vi "RT Loop - Acquisition and Logging.vi"(8 "error in (no error)":errorcluster, 9 "Acquisition and Logging Configuration":T1={"Data Rate (Hz)"=1.0, "Samples per Read"=0, "Number of Reads to Save"=0, "Data File Name"="", "TDMS Properties"=[], "Number of Channels"=4, "Channel Scale Array"=[0.0, 0.0, 0.0, 0.0], "Channel Names"=[], "Trigger - RMS Value"=0.0, "Trigger - Channel"=0, "Trigger - Time (Minute)"=0, "Enable RMS Trigger"=FALSE, "Enable Time Trigger"=FALSE, "Always Log"=FALSE}, 10 "Acquisition and Logging Queue":refnum<queue>, 11 "Message Queue":refnum<queue>) -> ()   [LabVIEW 2022 SP3]
uses:
  support/Message Queue/Message Cluster.ctl
  controls/Acquisition and Logging Configuration.ctl
  controls/TDMS Properties.ctl
  Globals/Global - Configuration Options.vi
  support/Message Queue/Message Queue.lvlib
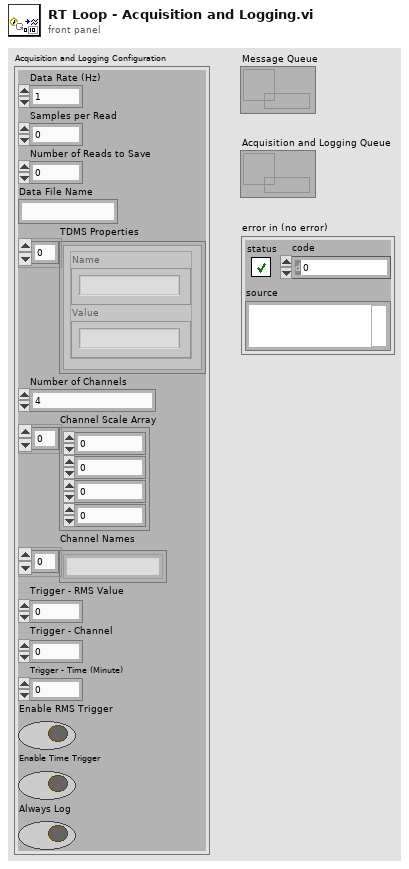
[diagram p1: front panel]
types:
  T1 = typedef "Acquisition and Logging Configuration.ctl" = cluster{"Data Rate (Hz)":dbl, "Samples per Read":i32, "Number of Reads to Save":i32, "Data File Name":string, "TDMS Properties":T2[], "Number of Channels":i32, "Channel Scale Array":dbl[], "Channel Names":string[], "Trigger - RMS Value":dbl, "Trigger - Channel":i32, "Trigger - Time (Minute)":i32, "Enable RMS Trigger":bool, "Enable Time Trigger":bool, "Always Log":bool}
  T2 = typedef "TDMS Properties.ctl" = cluster{"Name":string, "Value":string}
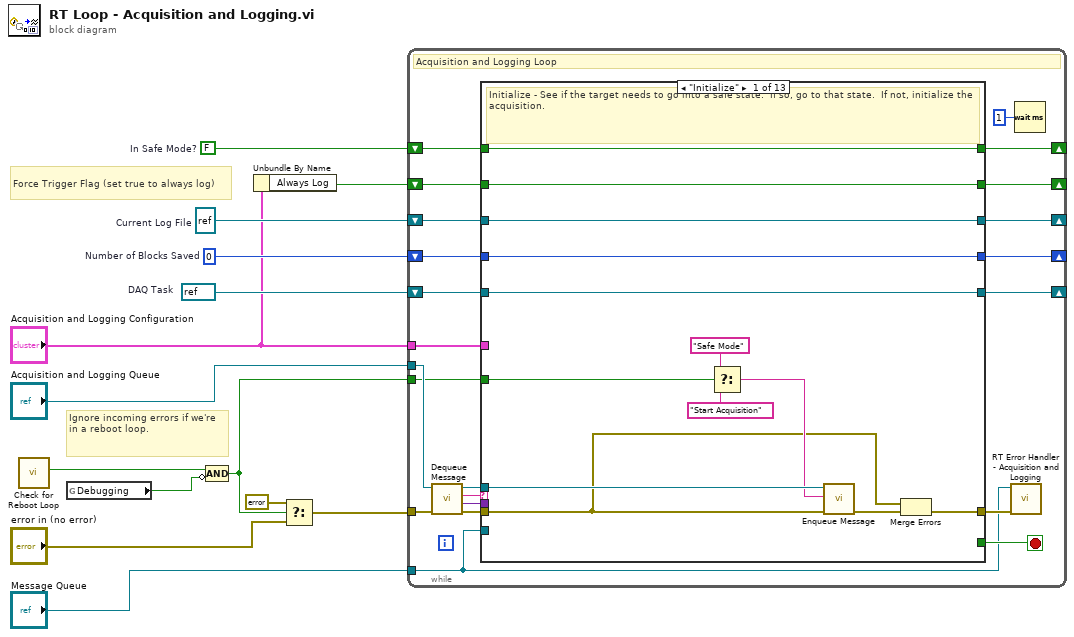
[diagram p0: block diagram]
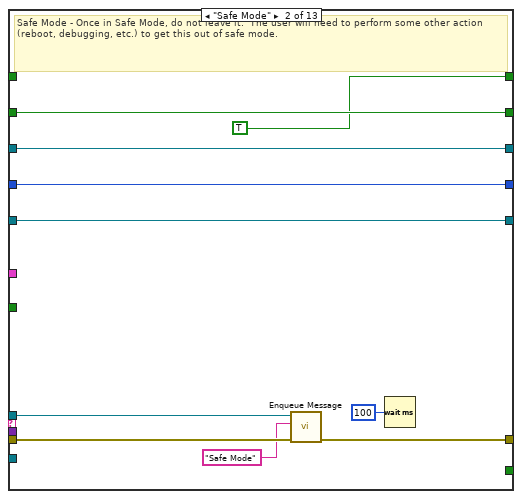
[diagram p2: hidden frame]
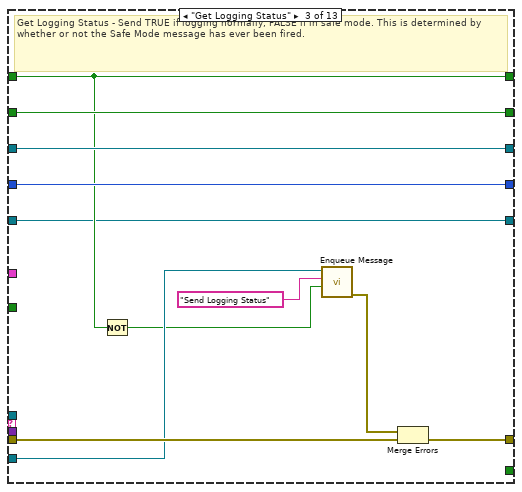
[diagram p3: hidden frame]
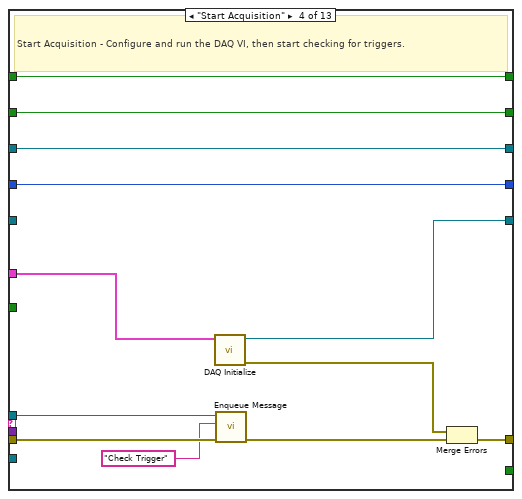
[diagram p4: hidden frame]
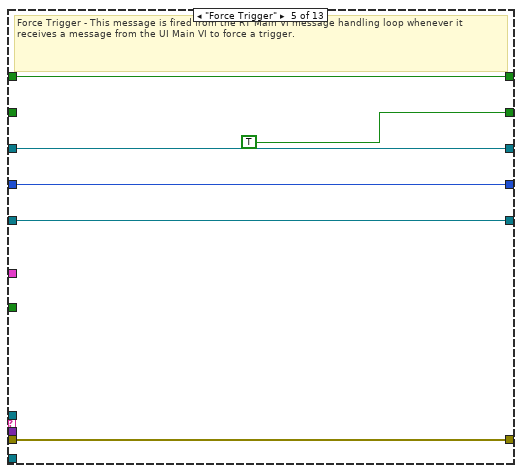
[diagram p5: hidden frame]
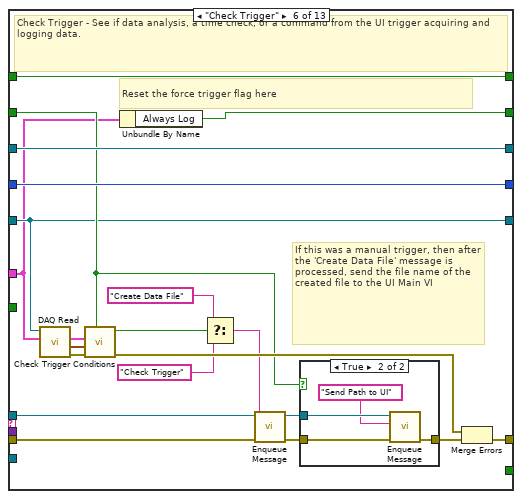
[diagram p6: hidden frame]
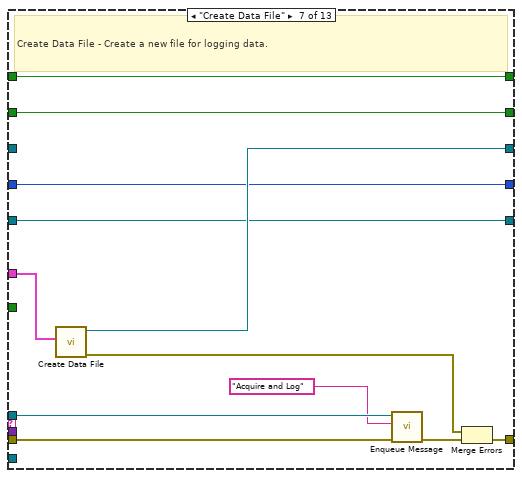
[diagram p8: hidden frame]
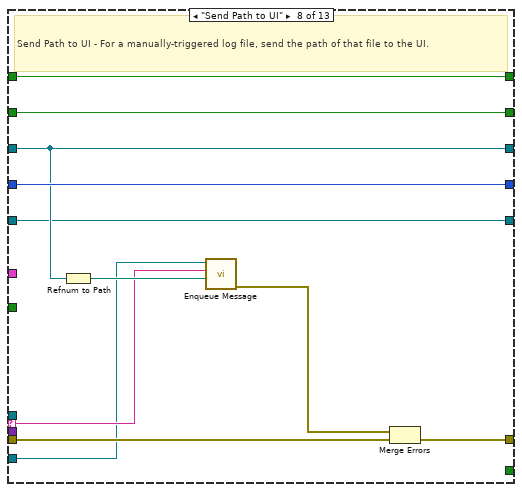
[diagram p9: hidden frame]
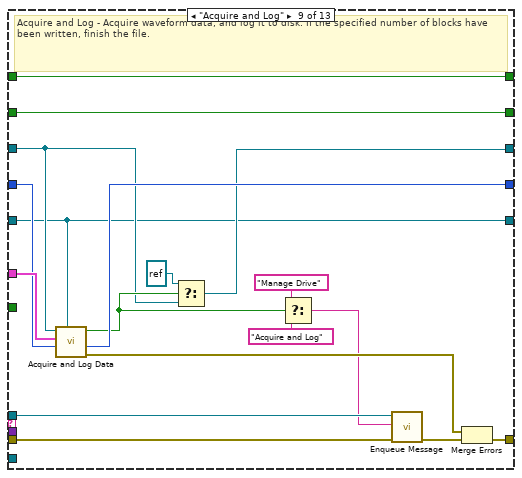
[diagram p10: hidden frame]
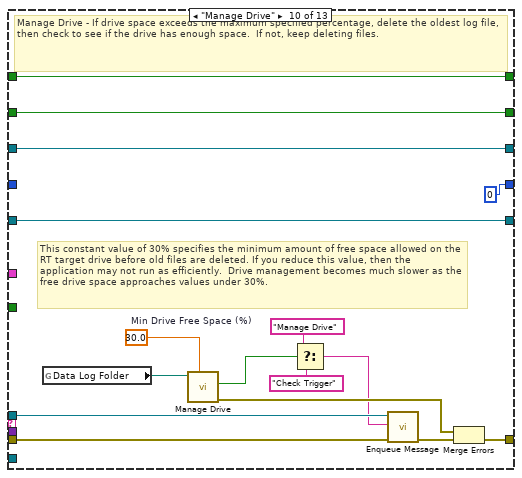
[diagram p11: hidden frame]
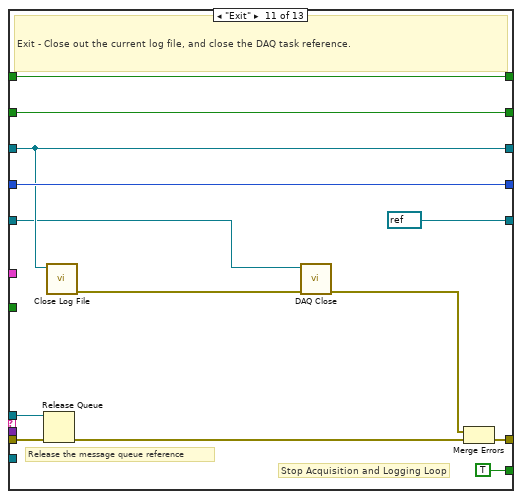
[diagram p12: hidden frame]
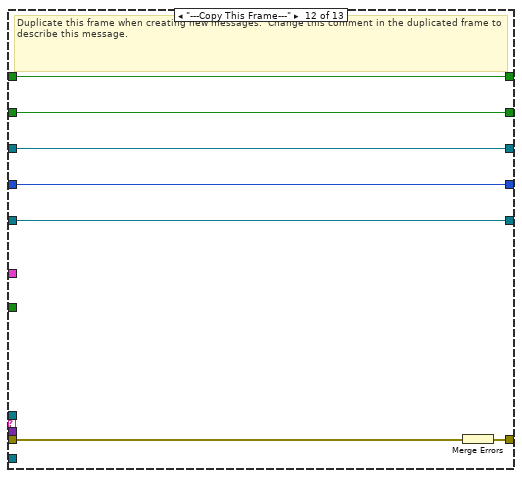
[diagram p13: hidden frame]
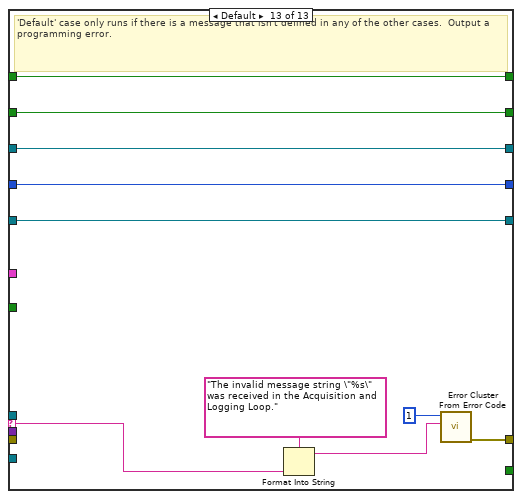
[diagram p14: hidden frame]
diagram:
  w9 = refnum<k21> refnum  # DAQ Task
  w10 = FALSE  # In Safe Mode?
  w11 = 0  # Number of Blocks Saved
  w12 = refnum<k34> refnum  # Current Log File
  # "Force Trigger Flag (set true to always log)"
  # "Ignore incoming errors if we're in a reboot loop."
  n1 = call "Check for Reboot Loop.vi"() -> ("Start in Safe Mode?"=w7:bool)  [unwired: 11 in]
  n2 = global read "Global - Configuration Options.vi" "Debugging"() -> (w8:bool)
  n3 = Compound Arithmetic op=AND(w7, invert w8) -> (w3:bool)
  n4 = Unbundle By Name("Acquisition and Logging Configuration") -> ("Always Log"=w2:bool)
  n5 = Select(t=errorcluster {"status"=FALSE, "code"=0, "source"=""}, s=w3, f="error in (no error)") -> (s? t:f=w4:errorcluster)
  n6 = while {
    tunnel: "Acquisition and Logging Queue" -> [w32]
    tunnel: "Message Queue" -> [w22]
    tunnel: "Acquisition and Logging Configuration" -> [w29]
    shift-right: [w27] -> _
    shift-left: w2 -> [w28]
    shift-right: [w25] -> _
    shift-left: w12 -> [w26]
    shift-right: [w23] -> _
    shift-left: w11 -> [w24]
    tunnel: w4 -> [w21]
    shift-right: [w19] -> _
    shift-left: w10 -> [w20]
    shift-right: [w17] -> _
    shift-left: w9 -> [w18]
    tunnel: w3 -> [w16]
    stop <- w36 stop-if-true
    # "Acquisition and Logging Loop"
    n7 = call "Dequeue Message.vi"("error in (no error)"=w21, "Message Queue"=w32) -> ("error out"=w35:errorcluster, "Message Data"=w33:variant, "Message"=w34:string, "dup Message Queue"=w30:refnum<queue>)  [unwired: 6 in]
    n8 = case "Message Cases" shown="\"Initialize\"" w34 {
      selector: w34 -> [_ _ _ _ _ _ _ w132 _ _ _ _ w200]
      tunnel: w30 -> [w47 w58 _ w77 _ w103 w123 _ w152 w167 w184 _ _]
      tunnel: w35 -> [w38 w59 w70 w82 w88 w109 w126 w137 w155 w171 w180 w191 _]
      tunnel: [w48 w57 w65 w80 w88 w108 w125 w130 w154 w170 w181 w190 w198] -> w31
      tunnel: [_ _ _ _ _ _ _ _ _ _ TRUE _ _] -> w36
      tunnel: w33 -> [_ _ _ _ _ _ _ _ _ _ _ _ _]
      tunnel: w29 -> [_ _ _ w81 _ w90 w120 _ w150 _ _ _ _]
      tunnel: w28 -> [w43 w56 w69 w75 _ w93 w121 w136 w151 w160 w179 w189 w196]
      tunnel: [w43 w56 w69 w75 TRUE ("Force Trigger Flag") w89 w121 w136 w151 w160 w179 w189 w196] -> w27
      tunnel: w26 -> [w42 w55 w68 w74 w87 w98 _ w134 w142 w156 w177 w188 w195]
      tunnel: [w42 w55 w68 w74 w87 w98 w118 w134 w141 w156 w177 w188 w195] -> w25
      tunnel: w24 -> [w41 w54 w67 w73 w85 w97 w117 w135 w145 _ w178 w187 w194]
      tunnel: [w41 w54 w67 w73 w85 w97 w117 w135 w144 0 ("Number of Blocks Saved") w178 w187 w194] -> w23
      tunnel: w22 -> [_ _ w66 _ _ _ _ w131 _ _ _ _ _]
      tunnel: w20 -> [w40 _ w61 w72 w84 w92 w116 w128 w139 w158 w176 w186 w193]
      tunnel: [w40 TRUE w61 w72 w84 w92 w116 w128 w139 w158 w176 w186 w193] -> w19
      tunnel: w18 -> [w39 w50 w60 _ w83 w91 w115 w127 w138 w157 w173 w185 w192]
      tunnel: [w39 w50 w60 w71 w83 w91 w115 w127 w138 w157 refnum<k21> refnum ("DAQ Task") w185 w192] -> w17
      tunnel: w16 -> [w37 _ _ _ _ _ _ _ _ _ _ _ _]
      frame "Initialize" {
        # "Initialize - See if the target needs to go into a safe state.  If so, go to that state.  If not, initialize the acquisition."
        n9 = Select(t="Safe Mode", s=w37, f="Start Acquisition") -> (s? t:f=w44:string)
        n10 = call "Enqueue Message.vi"("error in (no error)"=w38, "Message"=w44, "Message Queue"=w47) -> ("error out"=w49:errorcluster)  [unwired: 7 in, 1 out]
        n11 = Merge Errors(w38, w49) -> (w48:errorcluster)
      }
      frame "Safe Mode" {
        # "Safe Mode - Once in Safe Mode, do not leave it.  The user will need to perform some other action (reboot, debugging, etc.) to get this out of safe mode."
        n12 = call "Enqueue Message.vi"("error in (no error)"=w59, "Message"="Safe Mode", "Message Queue"=w58) -> ("error out"=w57:errorcluster)  [unwired: 7 in, 1 out]
        n13 = Wait (ms)(milliseconds to wait=u32 100) -> ()  [unwired: 1 out]
      }
      frame "Get Logging Status" {
        # "Get Logging Status - Send TRUE if logging normally, FALSE if in safe mode. This is determined by whether or not the Safe Mode message has ever been fired."
        n14 = Not(x=w61) -> (.not. x?=w63:bool)
        n15 = call "Enqueue Message.vi"("Message Data"=w63, "Message"="Send Logging Status", "Message Queue"=w66) -> ("error out"=w64:errorcluster)  [unwired: 7 in, 1 out]
        n16 = Merge Errors(w64, w70) -> (w65:errorcluster)
      }
      frame "Start Acquisition" {
        # "Start Acquisition - Configure and run the DAQ VI, then start checking for triggers."
        n17 = call "DAQ Initialize.vi"("Acquisition and Logging Configuration"=w81) -> ("error out"=w79:errorcluster, "DAQmx Task Name"=w71:refnum<k21>)  [unwired: 9 in]
        n18 = call "Enqueue Message.vi"("error in (no error)"=w82, "Message"="Check Trigger", "Message Queue"=w77) -> ("error out"=w78:errorcluster)  [unwired: 7 in, 1 out]
        n19 = Merge Errors(w79, w78) -> (w80:errorcluster)
      }
      frame "Force Trigger" {
        # "Force Trigger - This message is fired from the RT Main VI message handling loop whenever it receives a message from the UI Main VI to force a trigger."
      }
      frame "Check Trigger" {
        # "If this was a manual trigger, then after the 'Create Data File' message is processed, send the file name of the created file to the UI Main VI"
        # "Reset the force trigger flag here"
        # "Check Trigger - See if data analysis, a time check, or a command from the UI trigger acquiring and logging data."
        n20 = call "DAQ Read.vi"("Acquisition and Logging Configuration"=w90, "DAQmx Task Name"=w91) -> ("error out"=w106:errorcluster, "Waveform Data"=w105:waveform(dbl)[], "dup Acquisition and Logging Configuration"=w104:T1)  [unwired: 7 in]
        n21 = call "Check Trigger Conditions.vi"("Force Trigger?"=w93, "error in (no error)"=w106, "Waveform Data"=w105, "Acquisition and Logging Configuration"=w104) -> ("error out"=w107:errorcluster, "Trigger Condition Met?"=w102:bool)  [unwired: 6 in]
        n22 = Unbundle By Name(w90) -> ("Always Log"=w89:bool)
        n23 = Select(t="Create Data File", s=w102, f="Check Trigger") -> (s? t:f=w99:string)
        n24 = call "Enqueue Message.vi"("error in (no error)"=w109, "Message"=w99, "Message Queue"=w103) -> ("error out"=w96:errorcluster, "dup Message Queue"=w94:refnum<queue>)  [unwired: 7 in]
        n25 = case shown="True" w93 {
          tunnel: w96 -> [w110 w113]
          tunnel: [w110 w114] -> w95
          tunnel: w94 -> [_ w112]
          frame False {
          }
          frame True {
            n26 = call "Enqueue Message.vi"("error in (no error)"=w113, "Message"="Send Path to UI", "Message Queue"=w112) -> ("error out"=w114:errorcluster)  [unwired: 7 in, 1 out]
          }
        }
        n27 = Merge Errors(w107, w95) -> (w108:errorcluster)
      }
      frame "Create Data File" {
        # "Create Data File - Create a new file for logging data."
        n28 = call "Create Data File.vi"("Acquisition and Logging Configuration"=w120) -> ("error out"=w119:errorcluster, "TDMS File Reference"=w118:refnum<k34>)  [unwired: 9 in]
        n29 = call "Enqueue Message.vi"("error in (no error)"=w126, "Message"="Acquire and Log", "Message Queue"=w123) -> ("error out"=w124:errorcluster)  [unwired: 7 in, 1 out]
        n30 = Merge Errors(w119, w124) -> (w125:errorcluster)
      }
      frame "Send Path to UI" {
        # "Send Path to UI - For a manually-triggered log file, send the path of that file to the UI."
        n31 = Refnum to Path(1:w134) -> (0:w133:path)
        n32 = call "Enqueue Message.vi"("Message Data"=w133, "Message"=w132, "Message Queue"=w131) -> ("error out"=w129:errorcluster)  [unwired: 7 in, 1 out]
        n33 = Merge Errors(w129, w137) -> (w130:errorcluster)
      }
      frame "Acquire and Log" {
        # "Acquire and Log - Acquire waveform data, and log it to disk. If the specified number of blocks have been written, finish the file."
        n34 = call "Acquire and Log Data.vi"("DAQmx Task Name"=w138, "Number of Blocks Saved in"=w145, "Acquisition and Logging Configuration"=w150, "TDMS File Reference"=w142) -> ("error out"=w149:errorcluster, "Number of Blocks Saved out"=w144:i32, "Logging Complete?"=w143:bool)  [unwired: 5 in]
        n35 = Select(t=refnum<k34> refnum, s=w143, f=w142) -> (s? t:f=w141:refnum<k34>)
        n36 = Select(t="Manage Drive", s=w143, f="Acquire and Log") -> (s? t:f=w146:string)
        n37 = call "Enqueue Message.vi"("error in (no error)"=w155, "Message"=w146, "Message Queue"=w152) -> ("error out"=w153:errorcluster)  [unwired: 7 in, 1 out]
        n38 = Merge Errors(w149, w153) -> (w154:errorcluster)
      }
      frame "Manage Drive" {
        w169 = 30.0  # Min Drive Free Space (%)
        # "This constant value of 30% specifies the minimum amount of free space allowed on the RT target drive before old files are deleted. If you reduce this value, then the application may not run as efficiently.  Drive management becomes much slower as the free drive space approaches values under 30%."
        # "Manage Drive - If drive space exceeds the maximum specified percentage, delete the oldest log file, then check to see if the drive has enough space.  If not, keep deleting files."
        n39 = global read "Global - Configuration Options.vi" "Data Log Folder"() -> (w159:path)
        n40 = call "Manage Drive.vi"("Min Drive Free Space (%)"=w169, "Data Folder"=w159) -> ("error out"=w166:errorcluster, "Drive Space Below Limit"=w165:bool)  [unwired: 8 in]
        n41 = Select(t="Manage Drive", s=w165, f="Check Trigger") -> (s? t:f=w162:string)
        n42 = call "Enqueue Message.vi"("error in (no error)"=w171, "Message"=w162, "Message Queue"=w167) -> ("error out"=w168:errorcluster)  [unwired: 7 in, 1 out]
        n43 = Merge Errors(w166, w168) -> (w170:errorcluster)
      }
      frame "Exit" {
        # "Stop Acquisition and Logging Loop"
        # "Release the message queue reference"
        # "Exit - Close out the current log file, and close the DAQ task reference."
        n44 = Release Queue(queue=w184, error in (no error)=w180) -> (error out=w182:errorcluster)  [unwired: 1 in, 2 out]
        n45 = call "Close Log File.vi"("Log File"=w177) -> ("error out"=w175:errorcluster)  [unwired: 10 in]
        n46 = call "DAQ Close.vi"("error in (no error)"=w175, "DAQ Task"=w173) -> ("error out"=w174:errorcluster)  [unwired: 9 in]
        n47 = Merge Errors(w174, w182) -> (w181:errorcluster)
      }
      frame "---Copy This Frame---" {
        # "Duplicate this frame when creating new messages.  Change this comment in the duplicated frame to describe this message."
        n48 = Merge Errors(w191) -> (w190:errorcluster)
      }
      frame Default {
        # "'Default' case only runs if there is a message that isn't defined in any of the other cases.  Output a programming error."
        n49 = Format Into String(format string="The invalid message string \"%s\" was received in the Acquisition and Logging Loop." ("Unknown Message Error Text"), w200) -> (resulting string=w197:string)  [unwired: 2 in, 1 out]
        n50 = call <vilib>:"Error Cluster From Error Code.vi"("error message (\"\")"=w197, "error code (0)"=1) -> ("error out"=w198:errorcluster)  [unwired: 7 in]
      }
    }
    n51 = call "RT Error Handler - Acquisition and Logging.vi"("error in (no error)"=w31, "Message Queue"=w22) -> ()  [unwired: 9 in, 1 out]
    n52 = Wait (ms)(milliseconds to wait=u32 1) -> ()  [unwired: 1 out]
  }
